vi "Meas Get Record Section.vi"(5 "avg index ref":refnum<vi>, 7 "grp index ref":refnum<vi>, 8 "error in":errorcluster, 11 "record info":T1={"header path"=path "", "group id"=0, "average id"=0, "Time Stamp"=timestamp(0 s since 1904-01-01), "max samples"=0, "first sample"=0, "first smpl [%]"=-1.0, "kill viewer"=FALSE}) -> (0 "error out":errorcluster, 1 "record path":path, 2 "time [s]":ext[](array[numeric]), 3 "waveforms [V]":sgl[][](array[numeric]))   [LabVIEW 2018]
doc: "Reads desired section of the record defined in 'record info'. It will read the header file, it will parse it in order to find particular record in it, then it fetches desired portion of the sample data from binary sample file. Then it scales the data using scale factors from the header file."
uses:
  GUI/GUI Waveform Info.ctl
  octave/infolib.lvlibp/Private/Get key polymorph parts/GetI64.vi
  octave/infolib.lvlibp/Private/Get key polymorph parts/GetString.vi
  octave/infolib.lvlibp/Private/Get matrix polymorph parts/Get 1D String.vi
  octave/infolib.lvlibp/Private/Get matrix polymorph parts/Get 1D I64.vi
  octave/infolib.lvlibp/Private/Get matrix polymorph parts/Get 1D EXT.vi
  octave/infolib.lvlibp/Private/Get matrix polymorph parts/Get 2D EXT.vi
  octave/infolib.lvlibp
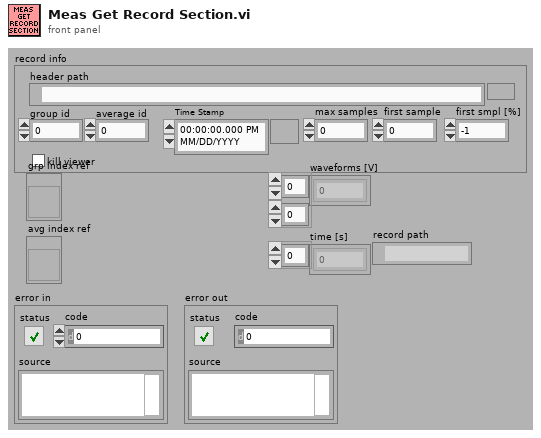
[diagram p1: front panel]
types:
  T1 = typedef "GUI Waveform Info.ctl" = cluster{"header path":path, "group id":i32, "average id":i32, "Time Stamp":timestamp, "max samples":i64, "first sample":i64, "first smpl [%]":dbl, "kill viewer":bool}
  T2 = typedef "MAT Type Representation.ctl" = enum16{"DBL", "SGL", "I32", "I16", "U16", "U8", "CDB", "CSG", "STR"}
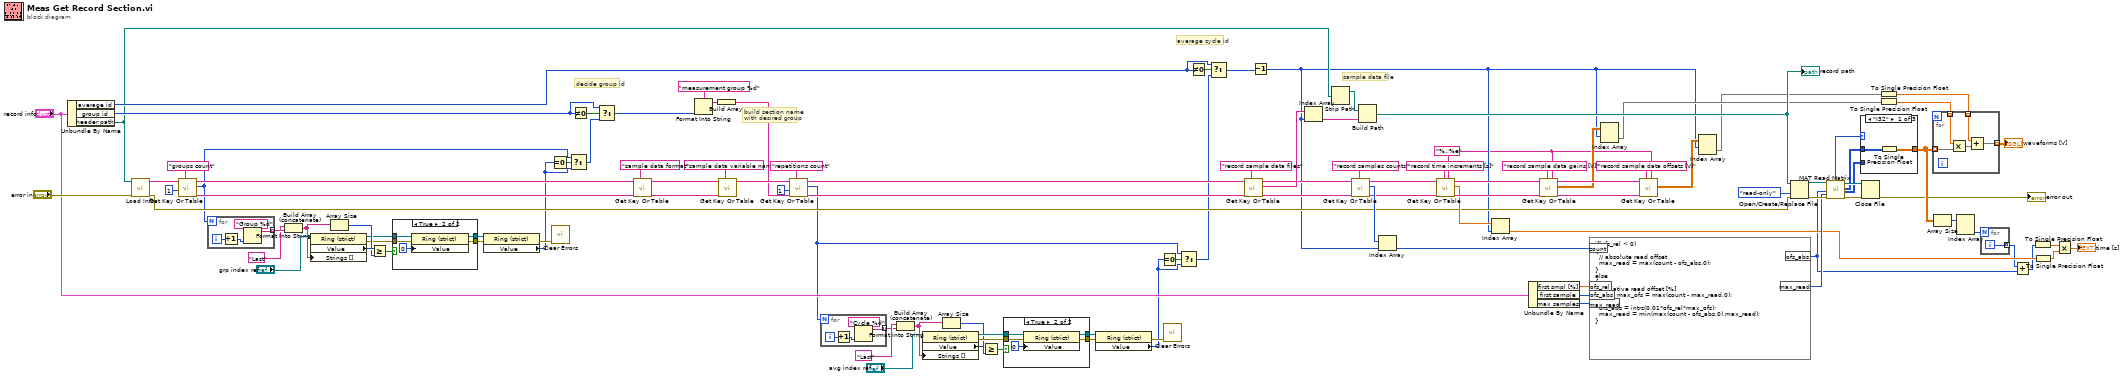
[diagram p0: block diagram]
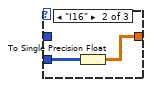
[diagram p4: hidden frame]
diagram:
  w1 = "%.;%e" ("format string (%_20f)")
  # "sample data file"
  # "average cycle id"
  # "decide group id"
  # "build section name\nwith desired group"
  n1 = Unbundle By Name("record info") -> ("average id"=w97:i32, "group id"=w104:i32, "header path"=w85:path)
  n2 = call "Load Info.vi"("error in"="error in", "filename"=w85) -> ("error out"=w43:errorcluster, "info data"=w108:string)  [unwired: 8 in]
  n3 = call-poly "Get Key Or Table.vi"("key description"="groups count", "numeric"=i64 1, "info data"=w108) -> ("sections out"=w77:string[], "value"=w6:i64, "info data out"=w82:string)  [unwired: 5 in, 1 out]
  n4 = for {
    N: w6 -> [_]
    tunnel: [w113] -> w32 mode=indexing
    i -> [w115]
    n5 = Increment(x=w115) -> (x+1=w112:i32)
    n6 = Format Into String(format string="Group %d", w112) -> (resulting string=w113:string)  [unwired: 2 in, 1 out]
  }
  n7 = Build Array (concatenate)("Last", w32) -> (w29:string[])
  n8 = property class="Ring (strict)"(reference="grp index ref", "Strings []"=w29) -> (reference out=w27:refnum<vi>, error out=w23:errorcluster, "Value"=w30:u16)  [unwired: 1 in]
  n9 = Array Size(array=w29) -> (size(s)=w28:i32)
  n10 = Greater Or Equal?(x=w30, y=w28) -> (x >= y?=w26:bool)
  n11 = case shown="True" w26 {
    tunnel: w27 -> [w117 w122]
    tunnel: [w117 w120] -> w25
    tunnel: [w116 w119] -> w24
    tunnel: w23 -> [w116 w118]
    frame False {
    }
    frame True {
      n12 = property class="Ring (strict)"(reference=w122, error in=w118, "Value"=u16 0) -> (reference out=w120:refnum<vi>, error out=w119:errorcluster)
    }
  }
  n13 = property class="Ring (strict)"(reference=w25, error in=w24) -> (error out=w22:errorcluster, "Value"=w8:u16)  [unwired: 1 out]
  n14 = Equal To 0?(x=w8) -> (x = 0?=w9:bool)
  n15 = call <vilib>:"Clear Errors.vi"("error in (no error)"=w22) -> ()  [unwired: 5 in, 2 out]
  n16 = Select(t=w6, s=w9, f=w8) -> (s? t:f=w7:i64)
  n17 = Not Equal To 0?(x=w104) -> (x != 0?=w105:bool)
  n18 = Select(t=w104, s=w105, f=w7) -> (s? t:f=w103:i64)
  n19 = call-poly "Get Key Or Table.vi"("key description"="sample data format", "sections"=w77, "info data"=w82) -> ("sections out"=w76:string[], "info data out"=w79:string)  [unwired: 5 in, 2 out]
  n20 = Format Into String(format string="measurement group %d", w103) -> (resulting string=w107:string)  [unwired: 2 in, 1 out]
  n21 = Build Array(w107) -> (w34:string[])
  n22 = call-poly "Get Key Or Table.vi"("key description"="sample data variable name", "sections"=w76, "info data"=w79) -> ("info data out"=w78:string)  [unwired: 5 in, 3 out]
  n23 = call-poly "Get Key Or Table.vi"("key description"="repetitions count", "sections"=w34, "numeric"=i64 1, "info data"=w78) -> ("sections out"=w102:string[], "value"=w2:i64, "info data out"=w101:string)  [unwired: 4 in, 1 out]
  n24 = for {
    N: w2 -> [_]
    tunnel: [w124] -> w11 mode=indexing
    i -> [w126]
    n25 = Increment(x=w126) -> (x+1=w123:i32)
    n26 = Format Into String(format string="Cycle %d", w123) -> (resulting string=w124:string)  [unwired: 2 in, 1 out]
  }
  n27 = Build Array (concatenate)("Last", w11) -> (w14:string[])
  n28 = property class="Ring (strict)"(reference="avg index ref", "Strings []"=w14) -> (reference out=w16:refnum<vi>, error out=w20:errorcluster, "Value"=w13:u16)  [unwired: 1 in]
  n29 = Array Size(array=w14) -> (size(s)=w15:i32)
  n30 = Greater Or Equal?(x=w13, y=w15) -> (x >= y?=w17:bool)
  n31 = case shown="True" w17 {
    tunnel: w16 -> [w128 w133]
    tunnel: [w128 w131] -> w18
    tunnel: [w127 w130] -> w19
    tunnel: w20 -> [w127 w129]
    frame False {
    }
    frame True {
      n32 = property class="Ring (strict)"(reference=w133, error in=w129, "Value"=u16 0) -> (reference out=w131:refnum<vi>, error out=w130:errorcluster)
    }
  }
  n33 = property class="Ring (strict)"(reference=w18, error in=w19) -> (error out=w21:errorcluster, "Value"=w3:u16)  [unwired: 1 out]
  n34 = Equal To 0?(x=w3) -> (x = 0?=w4:bool)
  n35 = call <vilib>:"Clear Errors.vi"("error in (no error)"=w21) -> ()  [unwired: 5 in, 2 out]
  n36 = Select(t=w2, s=w4, f=w3) -> (s? t:f=w5:i64)
  n37 = Not Equal To 0?(x=w97) -> (x != 0?=w98:bool)
  n38 = Select(t=w97, s=w98, f=w5) -> (s? t:f=w45:i64)
  n39 = call-poly "Get Key Or Table.vi"("key description"="record sample data files", "sections"=w102, "info data"=w101) -> ("sections out"=w93:string[], "value"=w95:string[], "info data out"=w92:string)  [unwired: 5 in, 1 out]
  n40 = Decrement(x=w45) -> (x-1=w38:i64)
  n41 = Index Array(array=w95, index=w38) -> (element=w83:string)
  n42 = Strip Path(path=w85) -> (stripped path=w84:path)  [unwired: 1 out]
  n43 = call-poly "Get Key Or Table.vi"("key description"="record samples counts", "sections"=w93, "info data"=w92) -> ("sections out"=w54:string[], "value"=w69:i64[], "info data out"=w53:string)  [unwired: 5 in, 1 out]
  n44 = Build Path(base path=w84, name or relative path=w83) -> (appended path=w65:path)
  "record path" <- w65
  n45 = Index Array(array=w69, index=w38) -> (element=w68:i64)
  n46 = call-poly "Get Key Or Table.vi"("format string (%_20f)"=w1, "key description"="record time increments [s]", "sections"=w54, "info data"=w53) -> ("sections out"=w51:string[], "value"=w46:ext[], "info data out"=w52:string)  [unwired: 4 in, 1 out]
  n47 = Index Array(array=w46, index=w38) -> (element=w44:ext)
  n48 = Unbundle By Name("record info") -> ("first smpl [%]"=w70:dbl, "first sample"=w71:i64, "max samples"=w67:i64)
  n49 = call-poly "Get Key Or Table.vi"("format string (%_20f)"=w1, "key description"="record sample data gains [V]", "sections"=w51, "info data"=w52) -> ("sections out"=w89:string[], "value"=w87:ext[][], "info data out"=w88:string)  [unwired: 4 in, 1 out]
  n50 = formula code="if(ofs_rel < 0)\n{\n  // absolute read offset\n  max_read = max(count - ofs_abs,0);\n}\nelse\n{\n  // relative read offset [%]\n  int32 max_ofs = max(count - max_read,0);\n  \n  ofs_abs = intrz(0.01*ofs_rel*max_ofs);\n  max_read = min(max(count - ofs_abs,0),max_read);\n}"("max_read"=w67, "count"=w68, "ofs_abs"=w71, "ofs_rel"=w70) -> ("ofs_abs"=w35:i64, "max_read"=w66:i64)
  n51 = Index Array(array=w87, index (row)=w38) -> (element=w59:ext[])  [unwired: 1 in]
  n52 = call-poly "Get Key Or Table.vi"("format string (%_20f)"=w1, "key description"="record sample data offsets [V]", "sections"=w89, "info data"=w88) -> ("value"=w86:ext[][])  [unwired: 4 in, 3 out]
  n53 = Index Array(array=w86, index (row)=w38) -> (element=w58:ext[])  [unwired: 1 in]
  n54 = Open/Create/Replace File(file path (use dialog)=w65, error in=w43, access (0:read/write)=enum16{"read/write", "read-only", "write-only"}."read-only") -> (refnum out=w73:refnum<file>, error out=w74:errorcluster)  [unwired: 3 in, 1 out]
  n55 = call "MAT Read Matrix.vi"("Ref Num"=w73, "first matrix column (0: first one)"=w35, "maximum matrix columns (-1: all)"=w66, "Error In"=w74) -> ("Representation"=w62:T2, "Dup Ref Num"=w63:refnum<file>, "I32"=w61:i32[][], "I16"=w60:i16[][], "error out"=w64:errorcluster)  [unwired: 3 in, 8 out]
  n56 = case shown="\"I32\"" w62 {
    tunnel: w61 -> [w135 _ _]
    tunnel: w60 -> [_ w137 _]
    tunnel: [w134 w136 _] -> w50
    frame "I32" {
      n57 = To Single Precision Float(number=w135) -> (single precision float=w134:sgl[][])
    }
    frame "I16" {
      n58 = To Single Precision Float(number=w137) -> (single precision float=w136:sgl[][])
    }
    frame Default {
    }
  }
  n59 = Close File(refnum=w63, error in=w64) -> (error out=→"error out":errorcluster)  [unwired: 1 out]
  n60 = To Single Precision Float(number=w58) -> (single precision float=w57:sgl[])
  n61 = To Single Precision Float(number=w59) -> (single precision float=w56:sgl[])
  n62 = for {
    tunnel: w50 -> [w142] mode=indexing
    tunnel: w56 -> [w141] mode=indexing
    tunnel: w57 -> [w139] mode=indexing
    tunnel: [w138] -> w41 mode=indexing
    n63 = Multiply(x=w141, y=w142) -> (x*y=w140:sgl[])
    n64 = Add(x=w139, y=w140) -> (x+y=w138:sgl[])
  }
  "waveforms [V]" <- w41
  n65 = Array Size(array=w50) -> (size(s)=w49:i32[])
  n66 = Index Array(array=w49) -> (element #2=w48:i32)  [unwired: 2 in, 1 out]
  n67 = for {
    N: w48 -> [_]
    tunnel: [w143] -> w37 mode=indexing
    i -> [w143]
  }
  n68 = Add(x=w37, y=w35) -> (x+y=w36:i64[])
  n69 = To Single Precision Float(number=w36) -> (single precision float=w47:sgl[])
  n70 = To Single Precision Float(number=w44) -> (single precision float=w39:sgl)
  n71 = Multiply(x=w47, y=w39) -> (x*y=→"time [s]":sgl[])
